vi "Tests_EventQueue.vi"() -> ()   [LabVIEW 2020]
panel:
  out "Register Error":errorcluster
  out "Destroy Queue Error":errorcluster
  out "Event Struct Error":errorcluster
  out "Time":u32
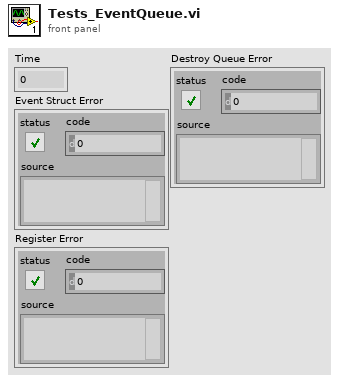
[diagram p1: front panel]
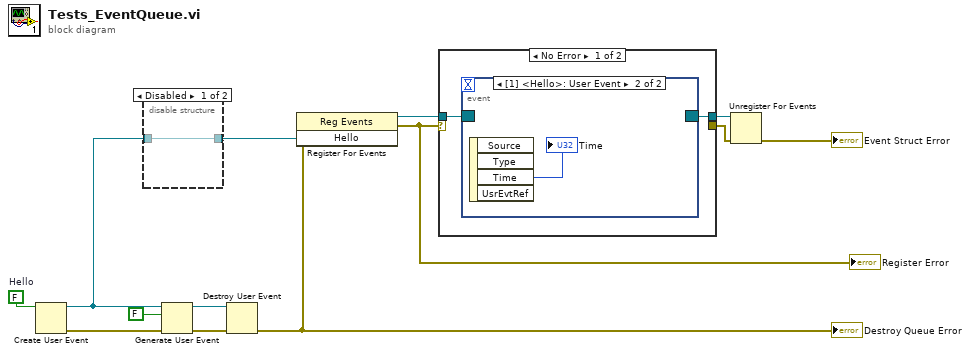
[diagram p0: block diagram]
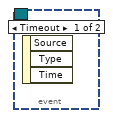
[diagram p3: hidden frame]
diagram:
  w13 = FALSE  # Hello
  n1 = Create User Event(user event datatype=w13) -> (user event=w3:refnum<user-event>, error out=w6:errorcluster)  [unwired: 1 in]
  n2 = disable-structure shown="Disabled" {
    disable-tunnel: w3 -> [w14 _]
    disable-tunnel: [w14 _] -> w2
    frame Disabled {
    }
    frame Enabled {
    }
  }
  n3 = Generate User Event(user event=w3, event data cluster=FALSE ("event data"), error in=w6) -> (user event out=w10:refnum<user-event>, error out=w7:errorcluster)  [unwired: 1 in]
  n4 = Destroy User Event(user event=w10, error in=w7) -> (error out=w4:errorcluster)
  "Destroy Queue Error" <- w4
  n5 = register-events(error in=w4, w2) -> (reference out=w12:refnum<event-registration>, error out=w1:errorcluster)  [unwired: 1 in]
  "Register Error" <- w1
  n6 = case shown="No Error" w1 {
    selector: w1 -> [_ w18]
    tunnel: w12 -> [w16 w19]
    tunnel: [w15 w19] -> w11
    tunnel: [_ w18] -> w9
    frame No Error {
      n7 = event shown="[1] <Hello>: User Event" {
        selector: w16 -> [_ _]
        dyn-events: [_ _] -> w15
        timeout: _ -> [_ _]
        event Timeout {
          n8 = event-data() -> ()  [unwired: 1 in, 3 out]
        }
        event User Event {
          n9 = event-data() -> ("Time"=→"Time":u32)  [unwired: 1 in, 3 out]
        }
      }
    }
    frame Error {
    }
  }
  n10 = Unregister For Events(event registration refnum=w11, error in=w9) -> (error out=→"Event Struct Error":errorcluster)
